vi "Init Panels.vi"(8 "error in (no error)":errorcluster, 11 "LV-Term App in":refnum<class "LV-Term App.lvclass">) -> (0 "error out":errorcluster, 3 "LV-Term App out":refnum<class "LV-Term App.lvclass">)   [LabVIEW 2020, in "LV-Term.lvlib" / "LV-Term App.lvclass"]
uses:
  LV-Term App.lvclass
  <vilib>/IlluminatedG/IG Terminal/Terminal/Terminal.lvclass
  C:/Program Files (x86)/National Instruments/LabVIEW 2020/vi.lib/IlluminatedG/IG OOPanel/OOPanel/Panel/Panel.lvclass
  LV-Term App.lvclass/LV-Term App.ctl
  <vilib>/IlluminatedG/IG OOPanel/OOPanel/Manager/Manager.lvclass
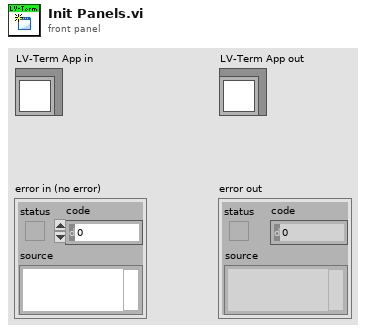
[diagram p1: front panel]
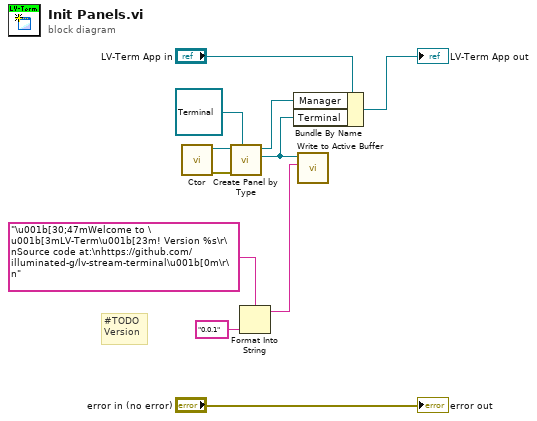
[diagram p0: block diagram]
diagram:
  # "#TODO\nVersion"
  n1 = call <vilib>:"Ctor.vi"() -> ("error out"=w8:errorcluster, "Manager out"=w10:refnum<class "Manager.lvclass">)  [unwired: 10 in]
  n2 = call <vilib>:"Create Panel by Type.vi"("Panel Type"=refnum<class "Terminal.lvclass"> refnum ("Terminal.lvlib:Terminal.lvclass"), "error in (no error)"=w8, "Manager in"=w10) -> ("Panel"=w4:refnum<class "Terminal.lvclass">, "Manager out"=w7:refnum<class "Manager.lvclass">)  [unwired: 6 in, 1 out]
  n3 = Format Into String(format string="\u001b[30;47mWelcome to \u001b[3mLV-Term\u001b[23m! Version %s\r\nSource code at:\nhttps://github.com/illuminated-g/lv-stream-terminal\u001b[0m\r\n" ("Data"), "0.0.1" ("input 1")) -> (resulting string=w1:string)  [unwired: 2 in, 1 out]
  n4 = Bundle By Name(cluster="LV-Term App in", "Manager"=w7, "Terminal"=w4) -> (→"LV-Term App out":refnum<class "LV-Term App.lvclass">)
  n5 = call <vilib>:"Write to Active Buffer.vi"("Data"=w1, "Terminal in"=w4) -> ()  [unwired: 8 in, 2 out]
  "error out" <- "error in (no error)"
